vi "IO_Control_New.vi"(6 "btnAbort":bool=TRUE, 8 "error in":errorcluster, 9 "output":refnum<k21>="Output", 10 "input":refnum<k21>="Input", 11 "Previous":bool[](array[boolean])) -> (0 "error out":errorcluster, 1 "lightCurtain":bool, 2 "On?":bool=TRUE, 3 "ThisArray":bool[](array[boolean]))   [LabVIEW 2015]
uses:
  <vilib>/DAQmx/read.llb/DAQmx Read (Digital 1D Bool NChan 1Samp 1Line).vi
  <vilib>/DAQmx/write.llb/DAQmx Write (Digital 1D Bool NChan 1Samp 1Line).vi
  <vilib>/DAQmx/miscellaneous.llb/DAQmx Fill In Error Info.vi
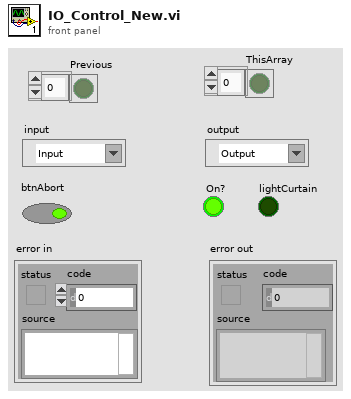
[diagram p1: front panel]
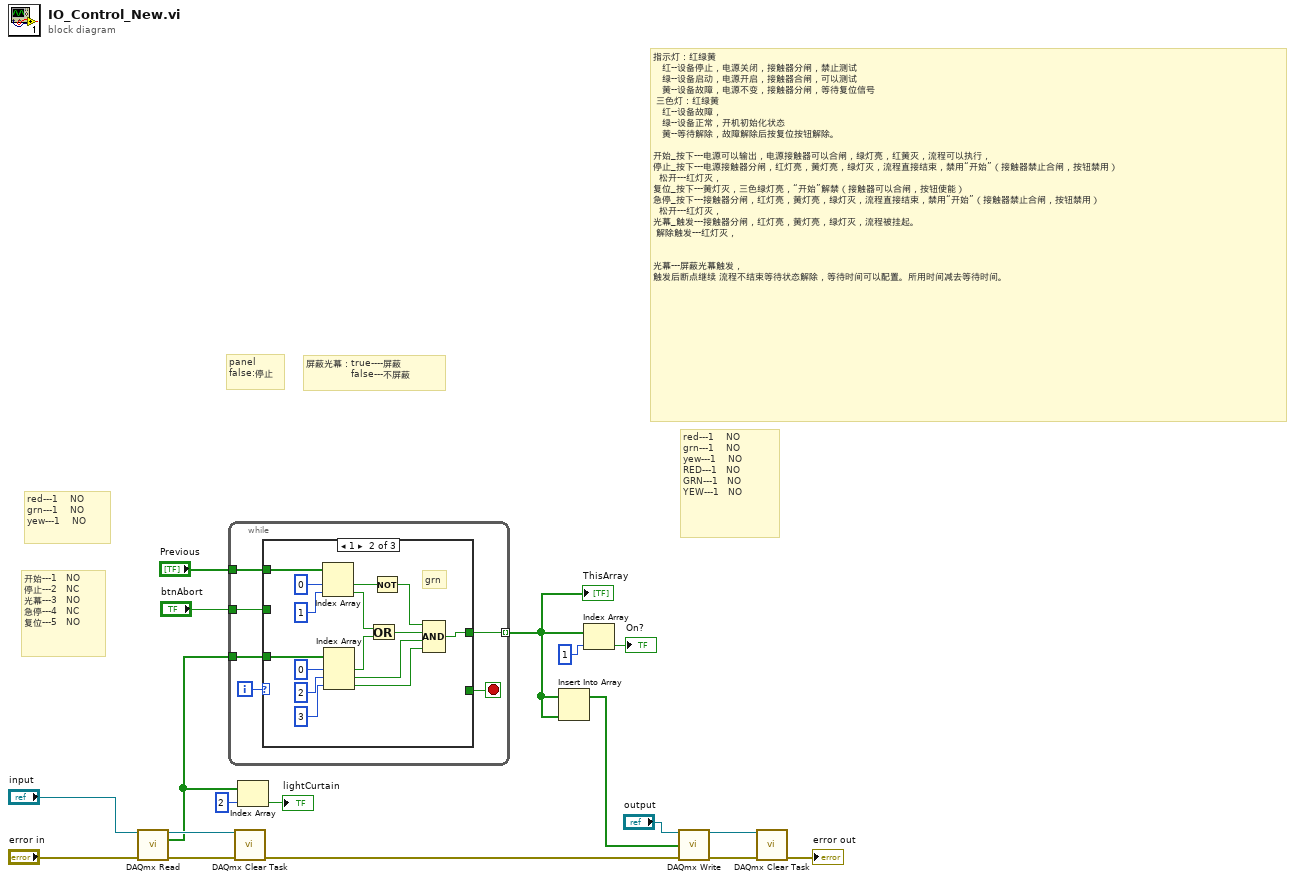
[diagram p0: block diagram]
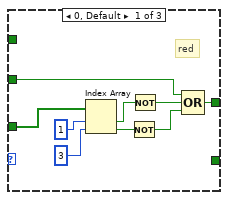
[diagram p2: hidden frame]
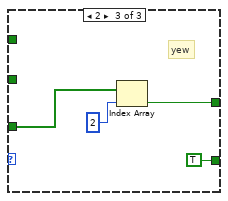
[diagram p3: hidden frame]
diagram:
  # "red---1    NO \ngrn---1    NO\nyew---1    NO"
  # "panel\nfalse:停止"
  # "屏蔽光幕：true----屏蔽\n               false---不屏蔽"
  # "指示灯：红绿黄\n\t\t\t红--设备停止，电源关闭，接触器分闸，禁止测试\n\t\t\t绿--设备启动，电源开启，接触器合闸，可以测试\n\t\t\t黄--设备故障，电源不变，接触器分闸，等待复位信号\n\t三色灯：红绿黄\n\t\t\t红--设备故障，\n\t\t\t绿--设备正常，开机初始化状态\n\t\t\t黄--等待解除，故障解除后按复位按钮解除。\n\n开始_按下---电源可以输出，电源接触器可以合闸，绿灯亮，红黄灭，流程可以执行，\n停止_按下---电源接触器分闸，红灯亮，黄灯亮，绿灯灭，流程直接结束，禁用“开始”（接触器禁止合闸，按钮禁用）\n\t 松开---红灯灭，\n复位_按下---黄灯灭，三色绿灯亮，“开始”解禁（接触器可以合闸，按钮使能）\n急停_按下---接触器分闸，红灯亮，黄灯亮，绿灯灭，流程直接结束，禁用“开始”（接触器禁止合闸，按钮禁用）\n\t 松开---红灯灭，\n光幕_触发---接触器分闸，红灯亮，黄灯亮，绿灯灭，流程被挂起。\n 解除触发---红灯灭，\n\n\n光幕---屏蔽光幕触发，\n触发后断点继续 流程不结束等待状态解除，等待时间可以配置。所用时间减去等待时间。"
  # "red---1    NO \ngrn---1    NO\nyew---1    NO\nRED---1   NO\nGRN---1   NO\nYEW---1   NO"
  # "开始---1   NO \n停止---2   NC\n光幕---3   NO\n急停---4   NC\n复位---5   NO"
  n1 = call-poly <vilib>:"DAQmx Read.vi"("task/channels in"="input", "error in"="error in") -> ("task out"=w16:refnum<k21>, "data"=w7:bool[], "error out"=w15:errorcluster)  [unwired: 11 in]
  n2 = while {
    tunnel: w7 -> [w24]
    tunnel: [w23] -> w1 mode=indexing
    tunnel: "Previous" -> [w21]
    tunnel: "btnAbort" -> [w20]
    i -> [w22]
    stop <- w19 stop-if-true
    n3 = case shown="1" w22 {
      tunnel: w24 -> [w25 w47 w52]
      tunnel: [w30 w39 w50] -> w23
      tunnel: w21 -> [_ w46 _]
      tunnel: w20 -> [w31 _ _]
      tunnel: [_ _ TRUE] -> w19
      frame 0, Default {
        # "red"
        n4 = Index Array(array=w25, index #1=1 ("index"), index #2=3 ("index")) -> (element #1=w32:bool, element #2=w27:bool)
        n5 = Not(x=w27) -> (.not. x?=w26:bool)
        n6 = Not(x=w32) -> (.not. x?=w29:bool)
        n7 = Compound Arithmetic op=OR(w31, w29, w26) -> (w30:bool)
      }
      frame 1 {
        # "grn"
        n8 = Index Array(array=w46, index #1=0 ("index"), index #2=1 ("index")) -> (element #1=w41:bool, element #2=w43:bool)
        n9 = Index Array(array=w47, index #1=0 ("index"), index #2=2 ("index"), index #3=3 ("index")) -> (element #1=w45:bool, element #2=w37:bool, element #3=w34:bool)
        n10 = Or(x=w43, y=w45) -> (x .or. y?=w40:bool)
        n11 = Not(x=w41) -> (.not. x?=w36:bool)
        n12 = Compound Arithmetic op=AND(w36, w40, w37, w34) -> (w39:bool)
      }
      frame 2 {
        # "yew"
        n13 = Index Array(array=w52, index=2) -> (element=w50:bool)
      }
    }
  }
  "ThisArray" <- w1
  n14 = call <vilib>:"DAQmx Clear Task.vi"("task in"=w16, "error in"=w15) -> ("error out"=w14:errorcluster)  [unwired: 13 in]
  n15 = Index Array(array=w7, index=2) -> (element=→"lightCurtain":bool)
  n16 = Insert Into Array(array=w1, new element=w1) -> (w6:bool[])  [unwired: 1 in]
  n17 = Index Array(array=w1, index=1) -> (element=→"On?":bool)
  n18 = call-poly <vilib>:"DAQmx Write.vi"("task/channels in"="output", "data"=w6, "error in"=w14) -> ("task out"=w8:refnum<k21>, "error out"=w10:errorcluster)  [unwired: 10 in, 1 out]
  n19 = call <vilib>:"DAQmx Clear Task.vi"("task in"=w8, "error in"=w10) -> ("error out"=→"error out":errorcluster)  [unwired: 13 in]
